vi "MGI Center from 3 Points (SGL).vi"(1 "Three Points":sgl[][](array[numeric])=[[0.0, 0.0, 0.0], [0.0, 0.0, 0.0], [0.0, 0.0, 0.0]]) -> (0 "Center":sgl[](array[numeric]))   [LabVIEW 2020]
doc: "Calculate the center of a circle based on three points on the circle.\n\nAuthored by David A. Moore\nsupport@mooregoodideas.com\nwww.mooregoodideas.com\n\nCopyright (c) 2010, Moore Good Ideas, Inc.\n\nAll rights reserved.\n\nRedistribution and use in source and binary forms, with or without modification, are permitted provided that the following conditions are met:\n\n * Redistributions of source code must retain the above copyright notice, this list of conditions and the following disclaimer.\n * Redistributions in binary form must reproduce the above copyright notice, this list of conditions and the following disclaimer in the documentation and/or other materials provided with the distribution.\n * Neither the name of Moore Good Ideas, Inc. nor the names of its contributors may be used to endorse or promote products derived from this software without specific prior written permission.\n\nTHIS SOFTWARE IS PROVIDED BY THE COPYRIGHT HOLDERS AND CONTRIBUTORS \"AS IS\" AND ANY EXPRESS OR IMPLIED WARRANTIES, INCLUDING, BUT NOT LIMITED TO, THE IMPLIED WARRANTIES OF MERCHANTABILITY AND FITNESS FOR A PARTICULAR PURPOSE ARE DISCLAIMED. IN NO EVENT SHALL THE COPYRIGHT OWNER OR CONTRIBUTORS BE LIABLE FOR ANY DIRECT, INDIRECT, INCIDENTAL, SPECIAL, EXEMPLARY, OR CONSEQUENTIAL DAMAGES (INCLUDING, BUT NOT LIMITED TO, PROCUREMENT OF SUBSTITUTE GOODS OR SERVICES; LOSS OF USE, DATA, OR PROFITS; OR BUSINESS INTERRUPTION) HOWEVER CAUSED AND ON ANY THEORY OF LIABILITY, WHETHER IN CONTRACT, STRICT LIABILITY, OR TORT (INCLUDING NEGLIGENCE OR OTHERWISE) ARISING IN ANY WAY OUT OF THE USE OF THIS SOFTWARE, EVEN IF ADVISED OF THE POSSIBILITY OF SUCH DAMAGE."
uses:
  <userlib>/_MGI/Matrix & Vector/MGI Calculate Vector Length/MGI Calculate Vector Length SGL.vi
  <userlib>/_MGI/Matrix & Vector/MGI Dot Product/MGI Dot Product SGL.vi
panel:
  # "x"
  # "y"
  # "z"
  # "y"
  # "z"
  # "x"
  # "p1"
  # "p2"
  # "p3"
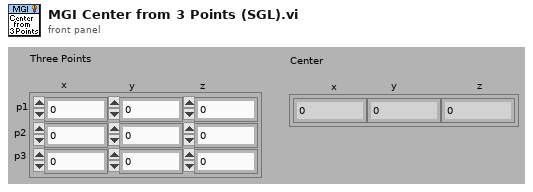
[diagram p1: front panel]
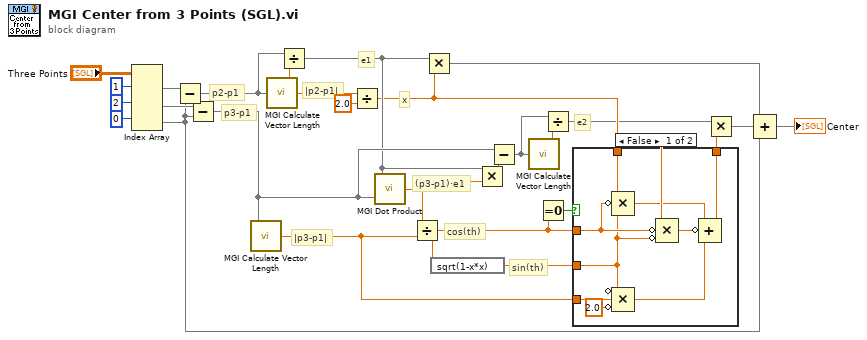
[diagram p0: block diagram]
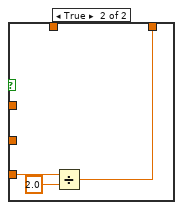
[diagram p2: hidden frame]
diagram:
  # "x"
  # "e2"
  # "sin(th)"
  # "cos(th)"
  # "(p3-p1)·e1"
  # "|p3-p1|"
  # "|p2-p1|"
  # "p3-p1"
  # "p2-p1"
  # "e1"
  n1 = Index Array(array="Three Points", index (row) #1=1 ("index (row)"), index (row) #2=2 ("index (row)"), index (row) #3=0 ("index (row)")) -> (element #1=w22:sgl[], element #2=w20:sgl[], element #3=w4:sgl[])  [unwired: 3 in]
  n2 = Subtract(x=w22, y=w4) -> (x-y=w21:sgl[])
  n3 = Subtract(x=w20, y=w4) -> (x-y=w16:sgl[])
  n4 = call-poly <userlib>:"MGI Calculate Vector Length.vi"("Vector"=w16) -> ("Distance"=w11:sgl)
  n5 = call-poly <userlib>:"MGI Calculate Vector Length.vi"("Vector"=w21) -> ("Distance"=w19:sgl)
  n6 = Divide(x=w21, y=w19) -> (x/y=w12:sgl[])
  n7 = Divide(x=w19, y=sgl 2.0) -> (x/y=w10:sgl)
  n8 = call-poly <userlib>:"MGI Dot Product.vi"("Y Vector"=w16, "X Vector"=w12) -> ("X * Y"=w13:sgl)
  n9 = Divide(x=w13, y=w11) -> (x/y=w1:sgl)
  n10 = Multiply(x=w12, y=w10) -> (x*y=w5:sgl[])
  n11 = expression code="sqrt(1-x*x)"(w1) -> (w9:sgl)
  n12 = Multiply(x=w12, y=w13) -> (x*y=w17:sgl[])
  n13 = Subtract(x=w16, y=w17) -> (x-y=w14:sgl[])
  n14 = call-poly <userlib>:"MGI Calculate Vector Length.vi"("Vector"=w14) -> ("Distance"=w15:sgl)
  n15 = Equal To 0?(x=w1) -> (x = 0?=w2:bool)
  n16 = Divide(x=w14, y=w15) -> (x/y=w8:sgl[])
  n17 = case shown="False" w2 {
    tunnel: w11 -> [w35 w38]
    tunnel: w10 -> [w33 _]
    tunnel: w1 -> [w32 _]
    tunnel: w9 -> [w31 _]
    tunnel: [w27 w36] -> w7
    frame False {
      n18 = Compound Arithmetic op=MULTIPLY(w33, invert w32, w31) -> (w30:sgl)
      n19 = Compound Arithmetic op=MULTIPLY(invert w31, w35, invert sgl 2.0 ("value")) -> (w29:sgl)
      n20 = Compound Arithmetic op=MULTIPLY(w33, invert w32, invert w31) -> (w28:sgl)
      n21 = Compound Arithmetic op=ADD(w30, invert w28, w29) -> (w27:sgl)
    }
    frame True {
      n22 = Divide(x=w38, y=sgl 2.0) -> (x/y=w36:sgl)
    }
  }
  n23 = Multiply(x=w8, y=w7) -> (x*y=w6:sgl[])
  n24 = Compound Arithmetic op=ADD(w5, w6, w4) -> (→"Center":sgl[])
